vi "IP Valid.vi"(1 "IP address":string) -> (0 "Valid?":bool)   [LabVIEW 2020]
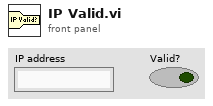
[diagram p1: front panel]
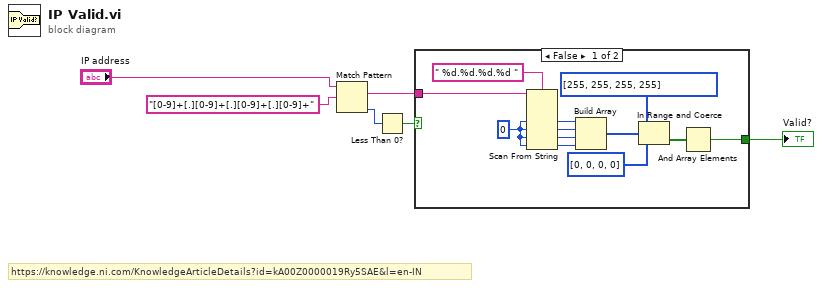
[diagram p0: block diagram]
diagram:
  # "https://knowledge.ni.com/KnowledgeArticleDetails?id=kA00Z0000019Ry5SAE&l=en-IN"
  n1 = Match Pattern(string="IP address", regular expression="[0-9]+[.][0-9]+[.][0-9]+[.][0-9]+") -> (match substring=w1:string, offset past match=w2:i32)  [unwired: 1 in, 2 out]
  n2 = Less Than 0?(x=w2) -> (x < 0?=w3:bool)
  n3 = case shown="False" w3 {
    tunnel: [w8 _] -> w4
    tunnel: w1 -> [w7 _]
    frame False {
      w17 = u16 0
      n4 = Scan From String(format string=" %d.%d.%d.%d ", input string=w7, default 1=w17, default 2=w17, default 3=w17, default 4=w17) -> (output 1=w16:u16, output 2=w15:u16, output 3=w14:u16, output 4=w13:u16)  [unwired: 2 in, 3 out]
      n5 = Build Array(w16, w15, w14, w13) -> (w12:u16[])
      n6 = In Range and Coerce(upper limit=u16[] [255, 255, 255, 255] ("lower limit"), x=w12, lower limit=u16[] [0, 0, 0, 0]) -> (In Range?=w9:bool[])  [unwired: 1 out]
      n7 = And Array Elements(Boolean array=w9) -> (logical AND=w8:bool)
    }
    frame True {
    }
  }
  "Valid?" <- w4
